vi "Generate ROIs.vi"() -> ()   [LabVIEW 2019]
uses:
  <vilib>/vision/NI_Vision_Development_Module.lvlib
panel:
  in  "Save ROI string data":path=path "C:/Users/ThymeLab/Desktop/Box12/rois_string"
  in  "Save ROI binary data":path=path "C:/Users/ThymeLab/Desktop/Box12/rois"
  out "roi data cluster":T1={[0, 0, 1088, 662], [{"Contour Type"=0, "ROI Type"=12, [74, 0, 155, 78, 89882]}, {"Contour Type"=0, "ROI Type"=12, [74, 79, 156, 157, 89882]}, {"Contour Type"=0, "ROI Type"=12, [75, 158, 156, 236, 89882]}, {"Contour Type"=0, "ROI Type"=12, [76, 236, 156, 314, 89882]}, {"Contour Type"=0, "ROI Type"=12, [76, 315, 157, 393, 89882]}, {"Contour Type"=0, "ROI Type"=12, [76, 394, 158, 472, 89882]}, {"Contour Type"=0, "ROI Type"=12, [77, 472, 158, 550, 89882]}, {"Contour Type"=0, "ROI Type"=12, [78, 551, 158, 629, 89882]}, {"Contour Type"=0, "ROI Type"=12, [155, 0, 236, 78, 89882]}, {"Contour Type"=0, "ROI Type"=12, [156, 79, 236, 157, 89882]}, {"Contour Type"=0, "ROI Type"=12, [156, 158, 237, 236, 89882]}, {"Contour Type"=0, "ROI Type"=12, [156, 236, 238, 314, 89882]}, {"Contour Type"=0, "ROI Type"=12, [157, 315, 238, 393, 89882]}, {"Contour Type"=0, "ROI Type"=12, [158, 394, 238, 472, 89882]}, {"Contour Type"=0, "ROI Type"=12, [158, 473, 239, 551, 89882]}, {"Contour Type"=0, "ROI Type"=12, [158, 551, 240, 629, 89882]}, {"Contour Type"=0, "ROI Type"=12, [236, 0, 317, 78, 89882]}, {"Contour Type"=0, "ROI Type"=12, [236, 79, 318, 157, 89882]}, {"Contour Type"=0, "ROI Type"=12, [237, 158, 318, 236, 89882]}, {"Contour Type"=0, "ROI Type"=12, [238, 237, 318, 315, 89882]}, {"Contour Type"=0, "ROI Type"=12, [238, 315, 319, 393, 89882]}, {"Contour Type"=0, "ROI Type"=12, [238, 394, 320, 472, 89882]}, {"Contour Type"=0, "ROI Type"=12, [239, 473, 320, 551, 89882]}, {"Contour Type"=0, "ROI Type"=12, [240, 552, 320, 630, 89882]}, {"Contour Type"=0, "ROI Type"=12, [317, 0, 398, 78, 89882]}, {"Contour Type"=0, "ROI Type"=12, [318, 79, 398, 157, 89882]}, {"Contour Type"=0, "ROI Type"=12, [318, 158, 399, 236, 89882]}, {"Contour Type"=0, "ROI Type"=12, [318, 237, 400, 315, 89882]}, {"Contour Type"=0, "ROI Type"=12, [319, 316, 400, 394, 89882]}, {"Contour Type"=0, "ROI Type"=12, [320, 394, 400, 472, 89882]}, {"Contour Type"=0, "ROI Type"=12, [320, 473, 401, 551, 89882]}, {"Contour Type"=0, "ROI Type"=12, [320, 552, 402, 630, 89882]}, {"Contour Type"=0, "ROI Type"=12, [398, 1, 479, 79, 89882]}, {"Contour Type"=0, "ROI Type"=12, [398, 79, 480, 157, 89882]}, {"Contour Type"=0, "ROI Type"=12, [399, 158, 480, 236, 89882]}, {"Contour Type"=0, "ROI Type"=12, [400, 237, 480, 315, 89882]}, {"Contour Type"=0, "ROI Type"=12, [400, 316, 481, 394, 89882]}, {"Contour Type"=0, "ROI Type"=12, [400, 394, 482, 472, 89882]}, {"Contour Type"=0, "ROI Type"=12, [401, 473, 482, 551, 89882]}, {"Contour Type"=0, "ROI Type"=12, [402, 552, 482, 630, 89882]}, {"Contour Type"=0, "ROI Type"=12, [479, 1, 560, 79, 89882]}, {"Contour Type"=0, "ROI Type"=12, [480, 80, 560, 158, 89882]}, {"Contour Type"=0, "ROI Type"=12, [480, 158, 561, 236, 89882]}, {"Contour Type"=0, "ROI Type"=12, [480, 237, 562, 315, 89882]}, {"Contour Type"=0, "ROI Type"=12, [481, 316, 562, 394, 89882]}, {"Contour Type"=0, "ROI Type"=12, [482, 395, 562, 473, 89882]}, {"Contour Type"=0, "ROI Type"=12, [482, 473, 563, 551, 89882]}, {"Contour Type"=0, "ROI Type"=12, [482, 552, 564, 630, 89882]}, {"Contour Type"=0, "ROI Type"=12, [560, 1, 641, 79, 89882]}, {"Contour Type"=0, "ROI Type"=12, [560, 80, 642, 158, 89882]}, {"Contour Type"=0, "ROI Type"=12, [561, 158, 642, 236, 89882]}, {"Contour Type"=0, "ROI Type"=12, [562, 237, 642, 315, 89882]}, {"Contour Type"=0, "ROI Type"=12, [562, 316, 643, 394, 89882]}, {"Contour Type"=0, "ROI Type"=12, [562, 395, 644, 473, 89882]}, {"Contour Type"=0, "ROI Type"=12, [563, 474, 644, 552, 89882]}, {"Contour Type"=0, "ROI Type"=12, [564, 552, 644, 630, 89882]}, {"Contour Type"=0, "ROI Type"=12, [641, 1, 722, 79, 89882]}, {"Contour Type"=0, "ROI Type"=12, [642, 80, 722, 158, 89882]}, {"Contour Type"=0, "ROI Type"=12, [642, 159, 723, 237, 89882]}, {"Contour Type"=0, "ROI Type"=12, [642, 237, 724, 315, 89882]}, {"Contour Type"=0, "ROI Type"=12, [643, 316, 724, 394, 89882]}, {"Contour Type"=0, "ROI Type"=12, [644, 395, 724, 473, 89882]}, {"Contour Type"=0, "ROI Type"=12, [644, 474, 725, 552, 89882]}, {"Contour Type"=0, "ROI Type"=12, [644, 552, 726, 630, 89882]}, {"Contour Type"=0, "ROI Type"=12, [722, 1, 803, 79, 89882]}, {"Contour Type"=0, "ROI Type"=12, [722, 80, 804, 158, 89882]}, {"Contour Type"=0, "ROI Type"=12, [723, 159, 804, 237, 89882]}, {"Contour Type"=0, "ROI Type"=12, [724, 238, 804, 316, 89882]}, {"Contour Type"=0, "ROI Type"=12, [724, 316, 805, 394, 89882]}, {"Contour Type"=0, "ROI Type"=12, [724, 395, 806, 473, 89882]}, {"Contour Type"=0, "ROI Type"=12, [725, 474, 806, 552, 89882]}, {"Contour Type"=0, "ROI Type"=12, [726, 553, 806, 631, 89882]}, {"Contour Type"=0, "ROI Type"=12, [803, 2, 884, 80, 89882]}, {"Contour Type"=0, "ROI Type"=12, [804, 80, 884, 158, 89882]}, {"Contour Type"=0, "ROI Type"=12, [804, 159, 885, 237, 89882]}, {"Contour Type"=0, "ROI Type"=12, [804, 238, 886, 316, 89882]}, {"Contour Type"=0, "ROI Type"=12, [805, 316, 886, 394, 89882]}, {"Contour Type"=0, "ROI Type"=12, [806, 395, 886, 473, 89882]}, {"Contour Type"=0, "ROI Type"=12, [806, 474, 887, 552, 89882]}, {"Contour Type"=0, "ROI Type"=12, [806, 553, 888, 631, 89882]}, {"Contour Type"=0, "ROI Type"=12, [884, 2, 965, 80, 89882]}, {"Contour Type"=0, "ROI Type"=12, [884, 80, 966, 158, 89882]}, {"Contour Type"=0, "ROI Type"=12, [885, 159, 966, 237, 89882]}, {"Contour Type"=0, "ROI Type"=12, [886, 238, 966, 316, 89882]}, {"Contour Type"=0, "ROI Type"=12, [886, 317, 967, 395, 89882]}, {"Contour Type"=0, "ROI Type"=12, [886, 395, 968, 473, 89882]}, {"Contour Type"=0, "ROI Type"=12, [887, 474, 968, 552, 89882]}, {"Contour Type"=0, "ROI Type"=12, [888, 553, 968, 631, 89882]}, {"Contour Type"=0, "ROI Type"=12, [965, 2, 1046, 80, 89882]}, {"Contour Type"=0, "ROI Type"=12, [966, 81, 1046, 159, 89882]}, {"Contour Type"=0, "ROI Type"=12, [966, 159, 1047, 237, 89882]}, {"Contour Type"=0, "ROI Type"=12, [966, 238, 1048, 316, 89882]}, {"Contour Type"=0, "ROI Type"=12, [967, 317, 1048, 395, 89882]}, {"Contour Type"=0, "ROI Type"=12, [968, 396, 1048, 474, 89882]}, {"Contour Type"=0, "ROI Type"=12, [968, 474, 1049, 552, 89882]}, {"Contour Type"=0, "ROI Type"=12, [968, 553, 1050, 631, 89882]}]}
  in  "Options":T2={"Interpolation Type"=enum."Bilinear Fixed", "Destination Width"=0, "Destination Height"=0, "Fill Value"=0.0}
  in  "Define Corner":bool
  in  "num Y cells":dbl=8.0
  in  "num X cells":dbl=12.0
  in  "three points":dbl[][](array[numeric])=[[74.0, 0.0], [1046.0, 2.0], [1050.0, 632.0]]
  out "Image":T3(plugin-control)
  in  "Path to Image":path=path "C:/Users/ThymeLab/Desktop/Box12/Box12.png"
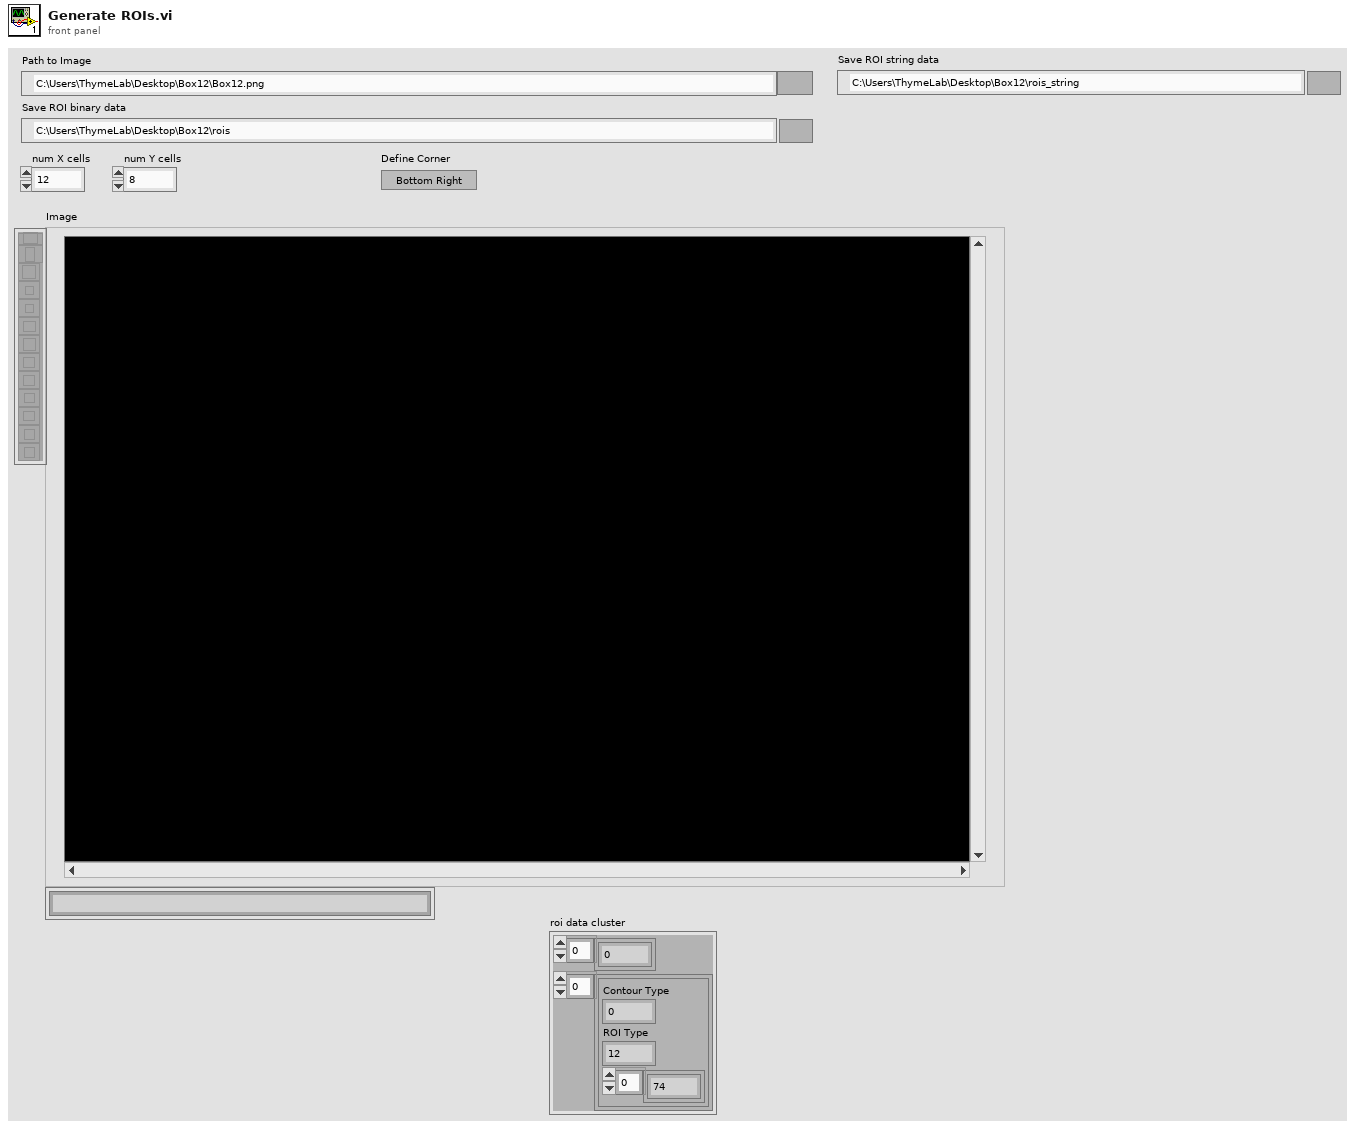
[diagram p1: front panel]
types:
  T1 = cluster{i32[], cluster{"Contour Type":u32, "ROI Type":u32, i32[]}[]}
  T2 = cluster{"Interpolation Type":enum32{"Zero Order", "Bilinear", "Quadratic", "Cubic", "Bilinear Fixed"}, "Destination Width":u32, "Destination Height":u32, "Fill Value":sgl}
  T3 = typedef "IMAQ Image.ctl" = refnum<image>
  T4 = enum16{"open", "replace", "create", "open or create", "replace or create", "replace or create with confirmation"}
  T5 = cluster{"Global Rectangle":i32[], "Contours":cluster{"Contour Type":u32, "ROI Type":u32, "Points":i32[]}[]}
  T6 = cluster{"Contour Type":u32, "ROI Type":u32, "Points":i32[]}[]
  T7 = cluster{"Contour Type":u32, "ROI Type":u32, "Points":i32[]}
  T8 = cluster{"Contour Type":u32, "ROI Type":u32, i32[]}
  T9 = cluster{"Contour Type":u32, "ROI Type":u32, i32[]}[]
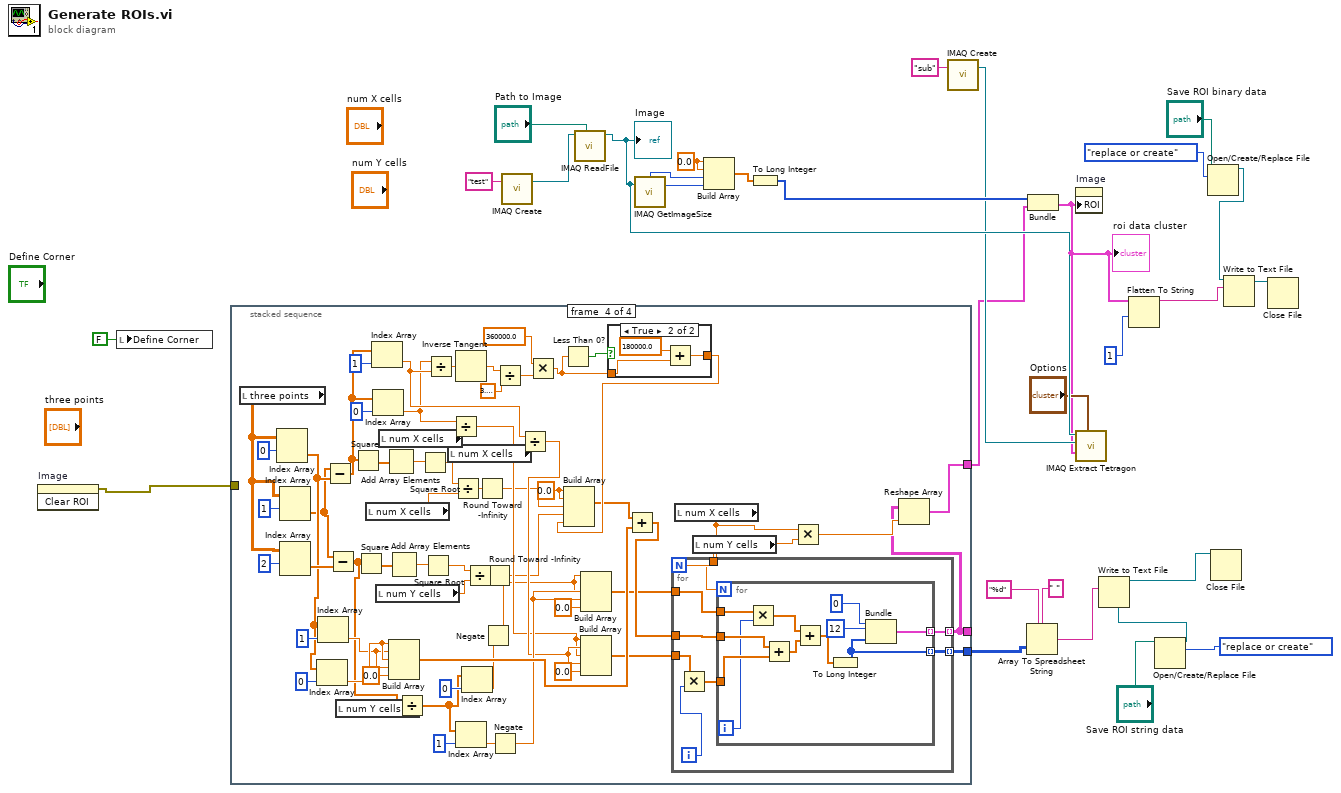
[diagram p0: block diagram]
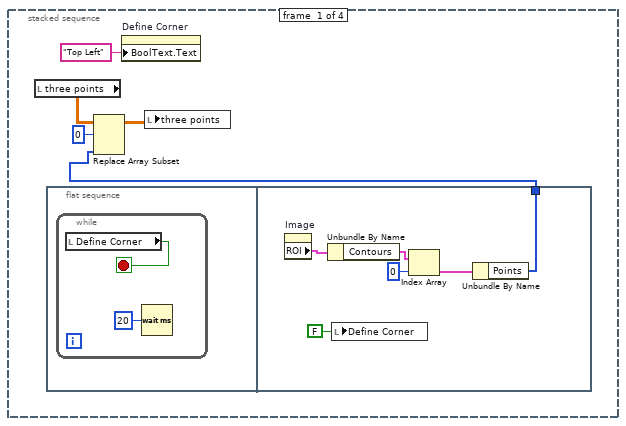
[diagram p2: hidden frame]
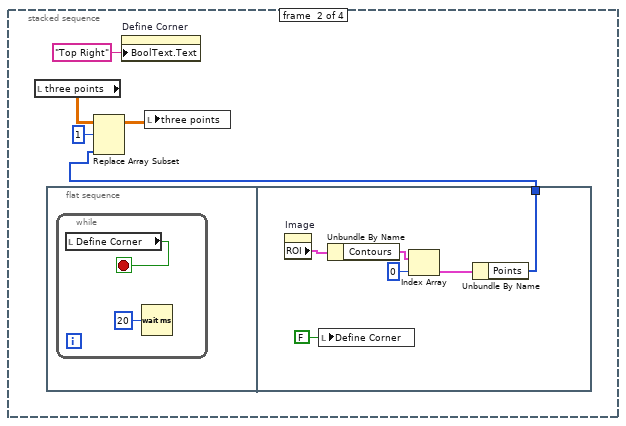
[diagram p3: hidden frame]
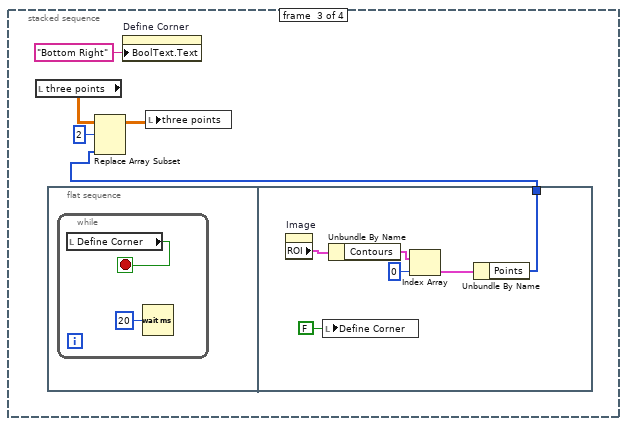
[diagram p4: hidden frame]
diagram:
  w26 = 0.0 ("element")
  n1 = invoke on="Image" class="ImageControl" method="Clear ROI"() -> (error out=w27:errorcluster)  [unwired: 3 in, 2 out]
  n2 = local write "Define Corner"(FALSE ("Define Corner")) -> ()
  n3 = stacked-sequence {
    tunnel: [_ _ _ w98] -> w3
    tunnel: w27 -> [_ _ _ _]
    tunnel: [_ _ _ w71] -> _
    tunnel: [_ _ _ w70] -> w1
    frame #0 {
      n4 = local read "three points"() -> (w33:dbl[][])
      n5 = flat-sequence {
        tunnel: [w39] -> w34
        frame #0 {
          n6 = while {
            stop <- w37 stop-if-true
            n7 = local read "Define Corner"() -> (w37:bool)
            n8 = Wait (ms)(milliseconds to wait=u32 20) -> ()  [unwired: 1 out]
          }
        }
        frame #1 {
          n9 = property on="Image" class="ImageControl"() -> ("ROI"=w43:T5)  [unwired: 2 in, 2 out]
          n10 = Unbundle By Name(w43) -> ("Contours"=w42:T6)
          n11 = local write "Define Corner"(FALSE ("Define Corner")) -> ()
          n12 = Index Array(array=w42, index=0) -> (element=w40:T7)
          n13 = Unbundle By Name(w40) -> ("Points"=w39:i32[])
        }
      }
      n14 = Replace Array Subset(array=w33, new element=w34, index (row)=0) -> (w32:dbl[][])  [unwired: 1 in]
      n15 = property on="Define Corner" class="Bool (strict)"("BoolText.Text"="Top Left" ("Boolean Text.Text")) -> ()  [unwired: 2 in, 2 out]
      n16 = local write "three points"(w32) -> ()
    }
    frame #1 {
      n17 = local read "three points"() -> (w46:dbl[][])
      n18 = flat-sequence {
        tunnel: [w52] -> w47
        frame #0 {
          n19 = while {
            stop <- w50 stop-if-true
            n20 = local read "Define Corner"() -> (w50:bool)
            n21 = Wait (ms)(milliseconds to wait=u32 20) -> ()  [unwired: 1 out]
          }
        }
        frame #1 {
          n22 = property on="Image" class="ImageControl"() -> ("ROI"=w56:T5)  [unwired: 2 in, 2 out]
          n23 = local write "Define Corner"(FALSE ("Define Corner")) -> ()
          n24 = Unbundle By Name(w56) -> ("Contours"=w55:T6)
          n25 = Index Array(array=w55, index=0) -> (element=w53:T7)
          n26 = Unbundle By Name(w53) -> ("Points"=w52:i32[])
        }
      }
      n27 = Replace Array Subset(array=w46, new element=w47, index (row)=1) -> (w45:dbl[][])  [unwired: 1 in]
      n28 = property on="Define Corner" class="Bool (strict)"("BoolText.Text"="Top Right" ("Boolean Text.Text")) -> ()  [unwired: 2 in, 2 out]
      n29 = local write "three points"(w45) -> ()
    }
    frame #2 {
      n30 = local read "three points"() -> (w59:dbl[][])
      n31 = flat-sequence {
        tunnel: [w65] -> w60
        frame #0 {
          n32 = while {
            stop <- w63 stop-if-true
            n33 = local read "Define Corner"() -> (w63:bool)
            n34 = Wait (ms)(milliseconds to wait=u32 20) -> ()  [unwired: 1 out]
          }
        }
        frame #1 {
          n35 = property on="Image" class="ImageControl"() -> ("ROI"=w69:T5)  [unwired: 2 in, 2 out]
          n36 = local write "Define Corner"(FALSE ("Define Corner")) -> ()
          n37 = Unbundle By Name(w69) -> ("Contours"=w68:T6)
          n38 = Index Array(array=w68, index=0) -> (element=w66:T7)
          n39 = Unbundle By Name(w66) -> ("Points"=w65:i32[])
        }
      }
      n40 = Replace Array Subset(array=w59, new element=w60, index (row)=2) -> (w58:dbl[][])  [unwired: 1 in]
      n41 = property on="Define Corner" class="Bool (strict)"("BoolText.Text"="Bottom Right" ("Boolean Text.Text")) -> ()  [unwired: 2 in, 2 out]
      n42 = local write "three points"(w58) -> ()
    }
    frame #3 {
      w107 = 0.0 ("element")
      n43 = local read "three points"() -> (w79:dbl[][])
      n44 = Index Array(array=w79, index (row)=0) -> (element=w97:dbl[])  [unwired: 1 in]
      n45 = Index Array(array=w79, index (row)=1) -> (element=w96:dbl[])  [unwired: 1 in]
      n46 = Index Array(array=w79, index (row)=2) -> (element=w126:dbl[])  [unwired: 1 in]
      n47 = Index Array(array=w97, index=0) -> (element=w106:dbl)
      n48 = Index Array(array=w97, index=1) -> (element=w105:dbl)
      n49 = Subtract(x=w96, y=w97) -> (x-y=w119:dbl[])
      n50 = Subtract(x=w96, y=w126) -> (x-y=w93:dbl[])
      n51 = local read "num Y cells"() -> (w110:dbl)
      n52 = Square(x=w119) -> (x^2=w131:dbl[])
      n53 = Square(x=w93) -> (x^2=w127:dbl[])
      n54 = local read "num X cells"() -> (w125:dbl)
      n55 = Index Array(array=w119, index=1) -> (element=w77:dbl)
      n56 = Index Array(array=w119, index=0) -> (element=w76:dbl)
      n57 = local read "num Y cells"() -> (w123:dbl)
      n58 = local read "num X cells"() -> (w111:dbl)
      n59 = Add Array Elements(numeric array=w131) -> (sum=w130:dbl)
      n60 = Add Array Elements(numeric array=w127) -> (sum=w128:dbl)
      n61 = Build Array(w106, w105, w106, w105, 0.0 ("element")) -> (w103:dbl[])
      n62 = Divide(x=w93, y=w110) -> (x/y=w90:dbl[])
      n63 = Square Root(x=w130) -> (sqrt(x)=w112:dbl)
      n64 = Square Root(x=w128) -> (sqrt(x)=w124:dbl)
      n65 = Divide(x=w76, y=w77) -> (x/y=w80:dbl)
      n66 = local read "num X cells"() -> (w88:dbl)
      n67 = Divide(x=w76, y=w111) -> (x/y=w86:dbl)
      n68 = Divide(x=w112, y=w125) -> (x/y=w114:dbl)
      n69 = Inverse Tangent(1:w80) -> (0:w81:dbl)
      n70 = Index Array(array=w90, index=1) -> (element=w94:dbl)
      n71 = Index Array(array=w90, index=0) -> (element=w89:dbl)
      n72 = Divide(x=w124, y=w123) -> (x/y=w113:dbl)
      n73 = Round Toward -Infinity(1:w114) -> (0:w73:dbl)
      n74 = Negate(x=w89) -> (-x=w85:dbl)
      n75 = Round Toward -Infinity(1:w113) -> (0:w72:dbl)
      n76 = Negate(x=w94) -> (-x=w92:dbl)
      n77 = Divide(x=w81, y=3.141592653589793) -> (x/y=w78:dbl)
      n78 = Divide(x=w77, y=w88) -> (x/y=w87:dbl)
      n79 = Multiply(x=360000.0, y=w78) -> (x*y=w116:dbl)
      n80 = Less Than 0?(x=w116) -> (x < 0?=w117:bool)
      n81 = Build Array(w85, w92, w85, w92, 0.0 ("element")) -> (w99:dbl[])
      n82 = Build Array(w86, w87, w86, w87, 0.0 ("element")) -> (w100:dbl[])
      n83 = case shown="True" w117 {
        tunnel: w116 -> [w153 w155]
        tunnel: [w153 w154] -> w115
        frame False {
        }
        frame True {
          n84 = Add(x=180000.0, y=w155) -> (x+y=w154:dbl)
        }
      }
      n85 = Build Array(w107, w107, w73, w72, w115) -> (w102:dbl[])
      n86 = Add(x=w102, y=w103) -> (x+y=w101:dbl[])
      n87 = local read "num X cells"() -> (w84:dbl)
      n88 = local read "num Y cells"() -> (w83:dbl)
      n89 = for {
        N: w84 -> [_]
        tunnel: w83 -> [w141]
        tunnel: w101 -> [w140]
        tunnel: w100 -> [w138]
        tunnel: w99 -> [w139]
        tunnel: [w135] -> w71 mode=indexing
        tunnel: [w134] -> w70 mode=indexing
        i -> [w137]
        n90 = Multiply(x=w138, y=w137) -> (x*y=w136:dbl[])
        n91 = for {
          N: w141 -> [_]
          tunnel: w140 -> [w150]
          tunnel: w139 -> [w148]
          tunnel: w136 -> [w149]
          tunnel: [w143] -> w135 mode=indexing
          tunnel: [w142] -> w134 mode=indexing
          i -> [w147]
          n92 = Multiply(x=w148, y=w147) -> (x*y=w144:dbl[])
          n93 = Add(x=w150, y=w149) -> (x+y=w145:dbl[])
          n94 = Add(x=w144, y=w145) -> (x+y=w146:dbl[])
          n95 = To Long Integer(number=w146) -> (32bit integer=w142:i32[])
          n96 = Bundle("Contour Type"=u32 0, "ROI Type"=u32 12, w142) -> (w143:T8)  [unwired: 1 in]
        }
      }
      n97 = Multiply(x=w84, y=w83) -> (x*y=w82:dbl)
      n98 = Reshape Array(w71, w82) -> (w98:T9)
    }
  }
  n99 = call "IMAQ Create"("Image Name"="test") -> ("New Image"=w29:T3)  [unwired: 4 in, 1 out]
  n100 = call "IMAQ ReadFile"("File Path"="Path to Image", "Image"=w29) -> ("Image Out"=w19:T3)  [unwired: 5 in, 4 out]
  "Image" <- w19
  n101 = call "IMAQ GetImageSize"("Image"=w19) -> ("Y Resolution"=w24:i32, "X Resolution"=w25:i32)  [unwired: 3 in, 1 out]
  n102 = Build Array(w26, w26, w25, w24) -> (w23:dbl[])
  n103 = To Long Integer(number=w23) -> (32bit integer=w22:i32[])
  n104 = call "IMAQ Create"("Image Name"="sub") -> ("New Image"=w18:T3)  [unwired: 4 in, 1 out]
  n105 = Array To Spreadsheet String(delimiter (Tab)=" ", array=w1, 3:"%d" ("format string")) -> (spreadsheet string=w5:string)
  n106 = Bundle(w22, w3) -> (w16:T1)  [unwired: 1 in]
  "roi data cluster" <- w16
  n107 = property on="Image" class="ImageControl"("ROI"=w16) -> ()  [unwired: 2 in, 2 out]
  n108 = call-poly "IMAQ Extract Tetragon"("Options"="Options", "ROI Descriptor"=w16, "Image Dst"=w18, "Image Src"=w19) -> ()  [unwired: 6 in, 2 out]
  n109 = Flatten To String(anything=w16, byte order (0:big-endian, network order)=1) -> (data string=w12:string)  [unwired: 2 in, 2 out]
  n110 = Open/Create/Replace File(file path (use dialog)="Save ROI string data", operation (0:open)=T4."replace or create") -> (refnum out=w8:refnum<file>)  [unwired: 4 in, 2 out]
  n111 = Write to Text File(file (use dialog)=w8, text=w5) -> (refnum out=w7:refnum<file>)  [unwired: 2 in, 2 out]
  n112 = Open/Create/Replace File(file path (use dialog)="Save ROI binary data", operation (0:open)=T4."replace or create") -> (refnum out=w13:refnum<file>)  [unwired: 4 in, 2 out]
  n113 = Close File(refnum=w7) -> ()  [unwired: 1 in, 2 out]
  n114 = Write to Text File(file (use dialog)=w13, text=w12) -> (refnum out=w11:refnum<file>)  [unwired: 2 in, 2 out]
  n115 = Close File(refnum=w11) -> ()  [unwired: 1 in, 2 out]
